vi "ReadIVBuffers.vi"(7 "GetCapacitors":bool, 8 "error in (no error)":errorcluster, 9 "Status":refnum<vi>, 10 "XYGraph Refnum":refnum<vi>, 11 "VISA Refnum in":refnum<visa-resource-name>) -> (0 "error out":errorcluster, 2 "CapacitanceInfos":T1[](array[typedef]), 3 "Array":dbl[][](array[numeric]))   [LabVIEW 2020]
uses:
  CapacitanceRecord.ctl
  Keithley 2600 Series/Keithley 2600 Series.lvlib
panel:
  out "Array 2":string[](array[string])
  out "error out 2":errorcluster
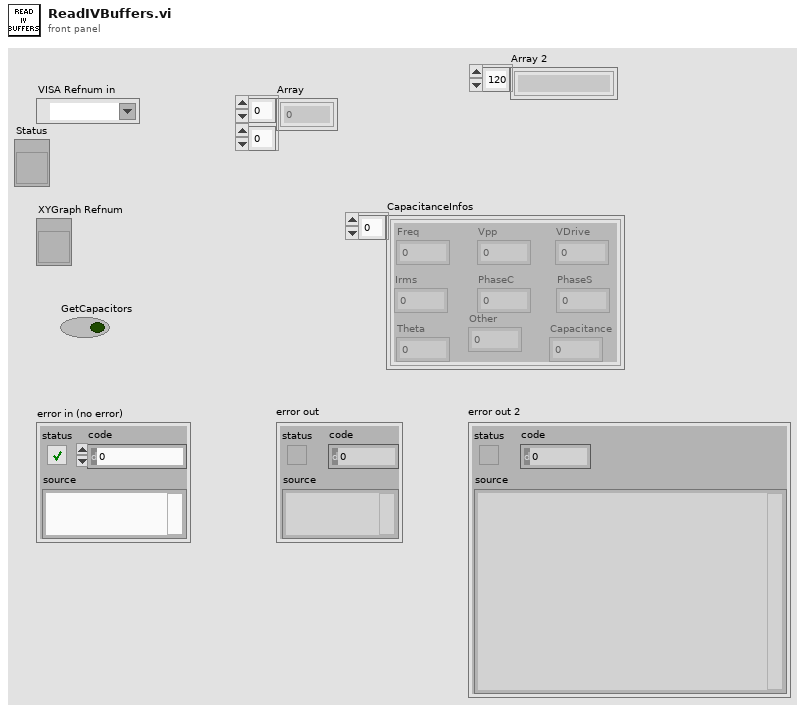
[diagram p1: front panel]
types:
  T1 = typedef "CapacitanceRecord.ctl" = cluster{"Freq":dbl, "Vpp":dbl, "PhaseS":dbl, "Irms":dbl, "PhaseC":dbl, "Theta":dbl, "VDrive":dbl, "Capacitance":dbl, "Other":dbl}
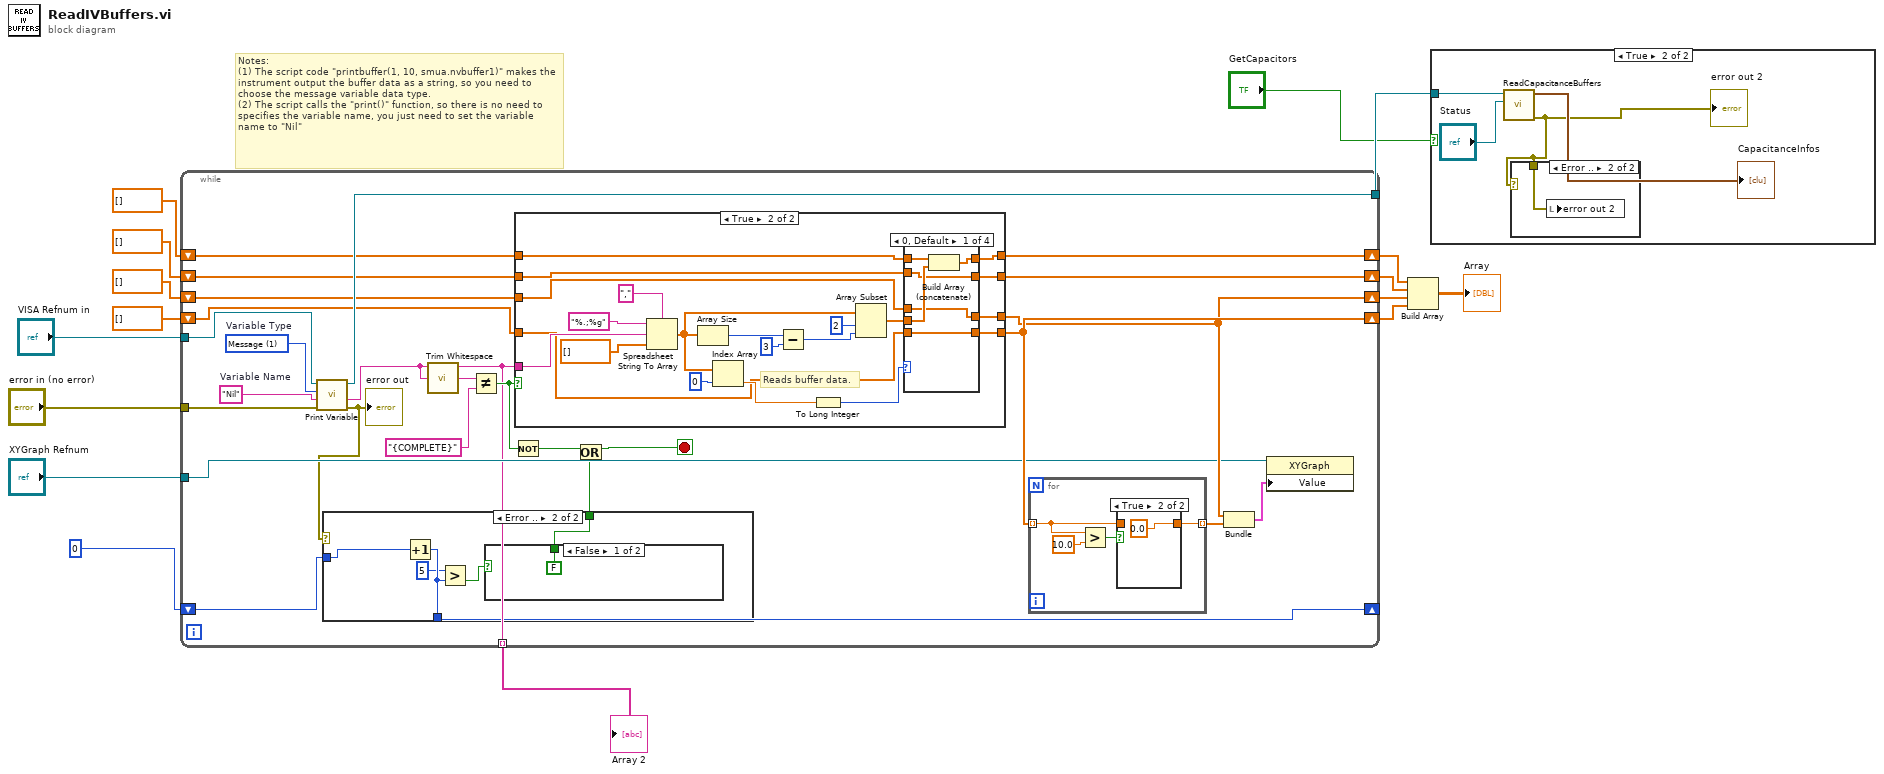
[diagram p0: block diagram]
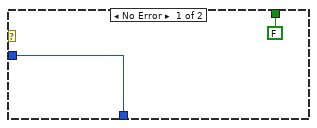
[diagram p4: hidden frame]
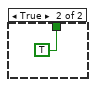
[diagram p5: hidden frame]
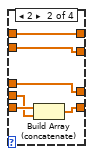
[diagram p8: hidden frame]
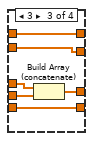
[diagram p9: hidden frame]
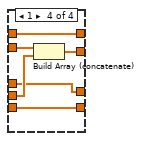
[diagram p10: hidden frame]
diagram:
  # "Notes: \n(1) The script code \"printbuffer(1, 10, smua.nvbuffer1)\" makes the instrument output the buffer data as a string, so you need to choose the message variable data type.\n(2) The script calls the \"print()\" function, so there is no need to specifies the variable name, you just need to set the variable name to \"Nil\""
  n1 = while {
    tunnel: "VISA Refnum in" -> [w40]
    tunnel: [w39] -> w4
    shift-right: [w34] -> w11
    shift-left: dbl[] [] ("array type (2D Dbl)") -> [w35]
    shift-right: [w24] -> w13
    shift-left: dbl[] [] ("array type (2D Dbl)") -> [w33]
    shift-right: [w38] -> w10
    shift-left: dbl[] [] ("array type (2D Dbl)") -> [w37]
    shift-right: [w25] -> w14
    shift-left: dbl[] [] ("array type (2D Dbl)") -> [w36]
    tunnel: "error in (no error)" -> [w28]
    tunnel: "XYGraph Refnum" -> [w23]
    tunnel: [w22] -> w2 mode=indexing
    shift-right: [w19] -> _
    shift-left: 0 -> [w20]
    stop <- w18 stop-if-true
    w42 = 1 items=["Number", "Message"]  # Variable Type
    w41 = "Nil"  # Variable Name
    n2 = call "Print Variable.vi"("error in (no error)"=w28, "Variable Name"=w41, "Variable Type (0: Number)"=w42, "VISA resource name"=w40) -> ("error out"=w21:errorcluster, "Message"=w22:string, "VISA resource name out"=w39:refnum<visa-resource-name>)  [unwired: 4 in, 1 out]
    "error out" <- w21
    n3 = case shown="Error .." w21 {
      tunnel: w20 -> [w44 w49]
      tunnel: [w44 w48] -> w19
      tunnel: [FALSE w45] -> w17
      frame No Error {
      }
      frame Error {
        n4 = Increment(x=w49) -> (x+1=w48:i32)
        n5 = Greater?(x=5, y=w48) -> (0:w47:bool)
        n6 = case shown="False" w47 {
          tunnel: [FALSE TRUE] -> w45
          frame False {
          }
          frame True {
          }
        }
      }
    }
    n7 = call <vilib>:"Trim Whitespace.vi"("string"=w22) -> ("trimmed string"=w32:string)  [unwired: 1 in]
    n8 = Not Equal?(x=w32, y="{COMPLETE}") -> (x != y?=w30:bool)
    n9 = Not(x=w30) -> (.not. x?=w29:bool)
    n10 = case shown="True" w30 {
      tunnel: w22 -> [_ w79]
      tunnel: [w61 w77] -> w38
      tunnel: w37 -> [w61 w76]
      tunnel: [w59 w74] -> w25
      tunnel: w36 -> [w59 w72]
      tunnel: w35 -> [w60 w71]
      tunnel: [w60 w70] -> w34
      tunnel: w33 -> [w58 w69]
      tunnel: [w58 w68] -> w24
      frame False {
      }
      frame True {
        # "Reads buffer data."
        n11 = Spreadsheet String To Array(delimiter (Tab)=",", format string="%.;%g", spreadsheet string=w79, array type (2D Dbl)=dbl[] []) -> (array=w65:dbl[])
        n12 = Array Size(array=w65) -> (size(s)=w64:i32)
        n13 = Index Array(array=w65, index=0) -> (element=w75:dbl)
        n14 = Subtract(x=w64, y=3) -> (x-y=w62:i32)
        n15 = To Long Integer(number=w75) -> (32bit integer=w73:i32)
        n16 = Array Subset(array=w65, index=2, length=w62) -> (w67:dbl[])
        n17 = case shown="0, Default" w73 {
          tunnel: [w86 w94 w100 w106] -> w77
          tunnel: w76 -> [w88 w94 w100 w106]
          tunnel: [w85 w89 w99 w102] -> w74
          tunnel: w67 -> [w87 w92 w96 w104]
          tunnel: w72 -> [w85 w93 w99 w102]
          tunnel: w71 -> [w84 w91 w98 w105]
          tunnel: [w84 w91 w98 w103] -> w70
          tunnel: w69 -> [w83 w90 w97 w101]
          tunnel: [w83 w90 w95 w101] -> w68
          frame 0, Default {
            n18 = Build Array (concatenate)(w88, w87) -> (w86:dbl[])
          }
          frame 2 {
            n19 = Build Array (concatenate)(w93, w92) -> (w89:dbl[])
          }
          frame 3 {
            n20 = Build Array (concatenate)(w97, w96) -> (w95:dbl[])
          }
          frame 1 {
            n21 = Build Array (concatenate)(w105, w104) -> (w103:dbl[])
          }
        }
      }
    }
    n22 = Or(x=w29, y=w17) -> (x .or. y?=w18:bool)
    n23 = for {
      tunnel: w25 -> [w53] mode=indexing
      tunnel: [w54] -> w26 mode=indexing
      n24 = Greater?(x=w53, y=10.0) -> (0:w55:bool)
      n25 = case shown="True" w55 {
        tunnel: [w56 0.0] -> w54
        tunnel: w53 -> [w56 _]
        frame False {
        }
        frame True {
        }
      }
    }
    n26 = Bundle("array type (2D Dbl)"=w24, w26) -> (w27:cluster{"array type (2D Dbl)":dbl[], dbl[]})  [unwired: 1 in]
    n27 = property class="XYGraph"(reference=w23, "Value"=w27) -> ()  [unwired: 1 in, 2 out]
  }
  "Array 2" <- w2
  n28 = Build Array(w10, w11, w13, w14) -> (→"Array":dbl[][])
  n29 = case shown="True" "GetCapacitors" {
    tunnel: w4 -> [_ w110]
    frame False {
    }
    frame True {
      n30 = call "ReadCapacitanceBuffers.vi"("Status"="Status", "VISA Refnum in"=w110) -> ("error out"=w107:errorcluster, "CapacitanceInfos"=→"CapacitanceInfos":T1[])  [unwired: 7 in, 1 out]
      "error out 2" <- w107
      n31 = case shown="Error .." w107 {
        tunnel: w107 -> [_ w111]
        frame No Error {
        }
        frame Error {
          n32 = local write "error out 2"(w111) -> ()
        }
      }
    }
  }
